vi "LoadFile.vi"(8 "content":string, 9 "name":string, 10 "HighSpeedEServer":refnum<k24>, 11 "error in (no error)":errorcluster) -> (3 "error out":errorcluster)   [LabVIEW 2019, in "UnderAutomation.Yaskawa.lvlib"]
uses:
  UnderAutomation.Yaskawa.lvlib
  C:/Users/fg/Documents/Yaskawa.vi/LabVIEW_2024/UnderAutomation.Yaskawa/lib/UnderAutomation.Yaskawa.dll
  LabVIEW_2024/UnderAutomation.Yaskawa/lib/UnderAutomation.Yaskawa.dll
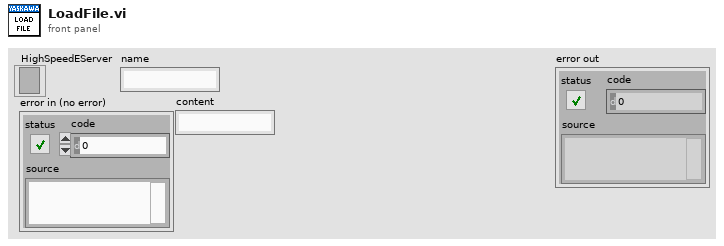
[diagram p1: front panel]
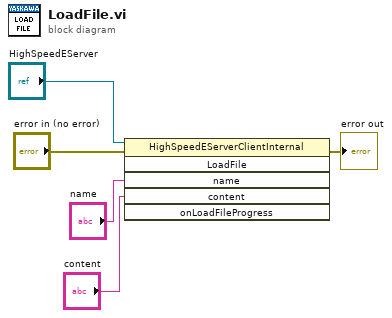
[diagram p0: block diagram]
diagram:
  n1 = invoke class="HighSpeedEServerClientInternal" method="LoadFile"(reference="HighSpeedEServer", error in="error in (no error)", "name"="name", "content"="content") -> (error out=→"error out":errorcluster)  [unwired: 2 in, 5 out]
